vi "Multiple_DT98xx_Ain_Async_PN.vi"(7 "Master board name":string="DT9816(00)", 8 "Samples per channel":u32=2000, 9 "Sampling rate (Hz)":dbl=20000.0, 10 "Slave channels to acquire":string="0,1,2,3,4,5", 11 "Master channels to acquire":string="0,1,2,3,4,5") -> (0 "Overall error":errorcluster, 2 "Slaves data":dbl[][][](array[numeric]), 3 "Master data":dbl[][](graph))   [LabVIEW 2022 SP3]
uses:
  Low levels/DtAinContinuous Folder/PolySubVIs/DtCreateAinChan.vi
  Low levels/DtAinContinuous Folder/PolySubVIs/DtOLTimingSetInput.vi
  <userlib>/LV-Link3/PolySubVIs/DtOLStartNormal.vi
  Low levels/DtAinContinuous Folder/PolySubVIs/DtCreateCtrRateChan.vi
panel:
  out "Slaves data (concat.)":dbl[][](graph)
  out "Master board index":i32
  out "Board names":string[](array[string])=["DT9816(00)", "DT9816(01)"]
  out "Number of boards":i32=2
  # "DEVICES MUST BE INTERCONNECTED AS FOLLOWS:\nMaster \"Counter 0 Out\" to Master \"Ext Clock\" and Slaves \"Ext Clock\""
  # "PN 18/10/2012"
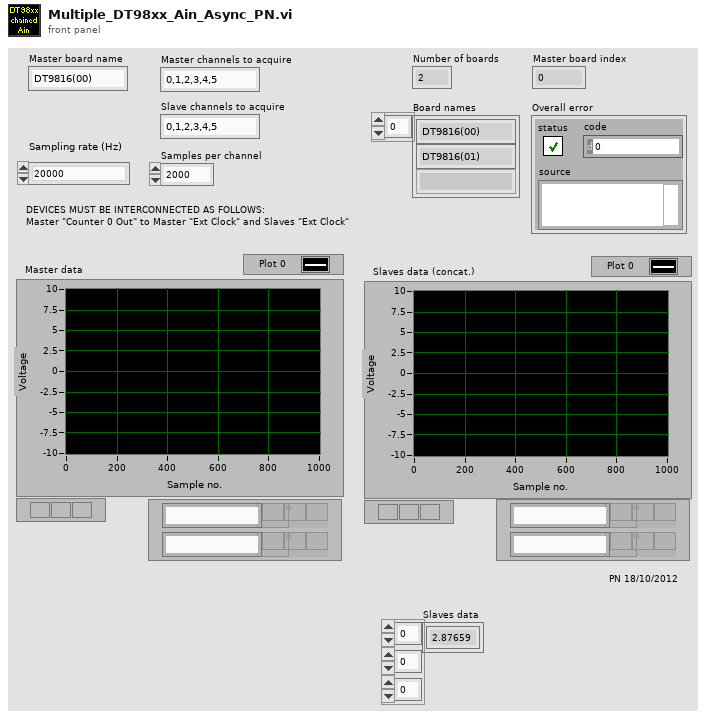
[diagram p1: front panel]
types:
  T1 = enum32{"Internal Clock", "External Clock", "No Timing"}
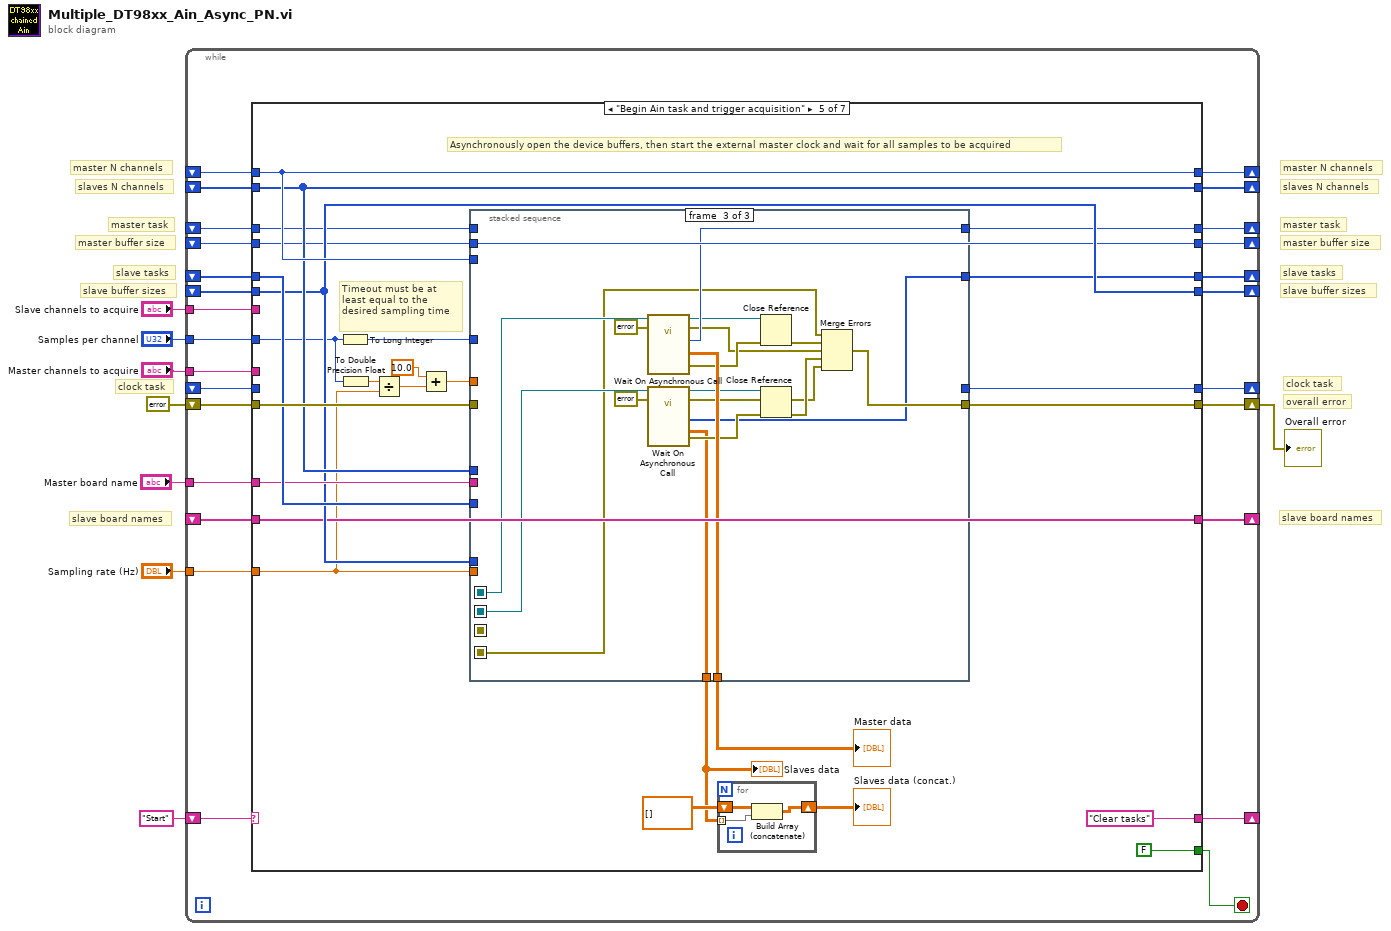
[diagram p0: block diagram]
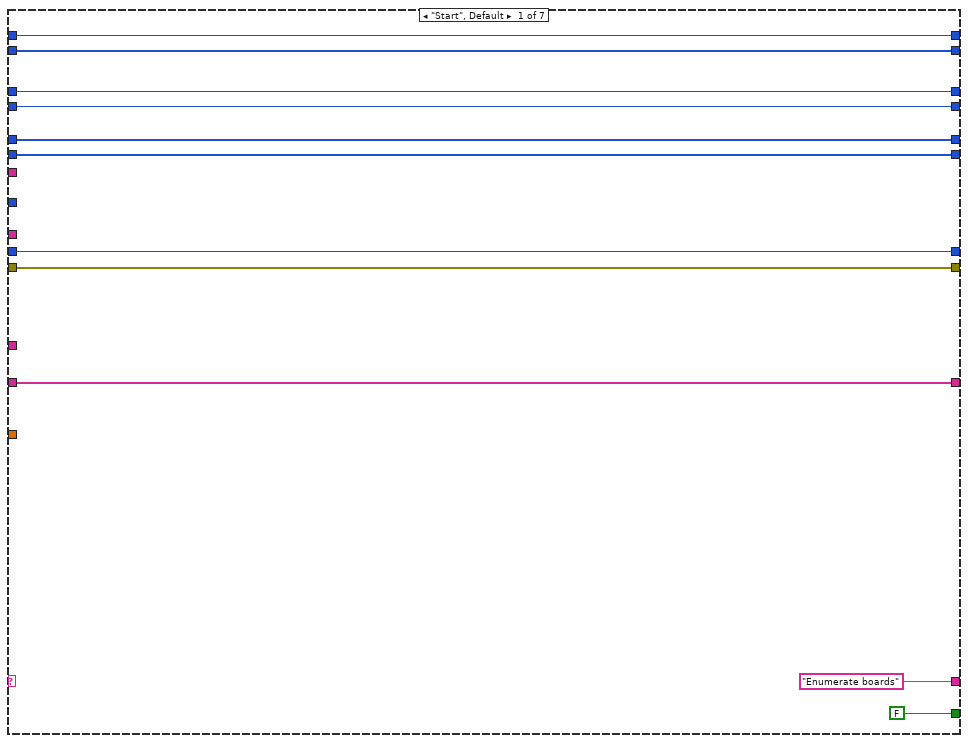
[diagram p2: hidden frame]
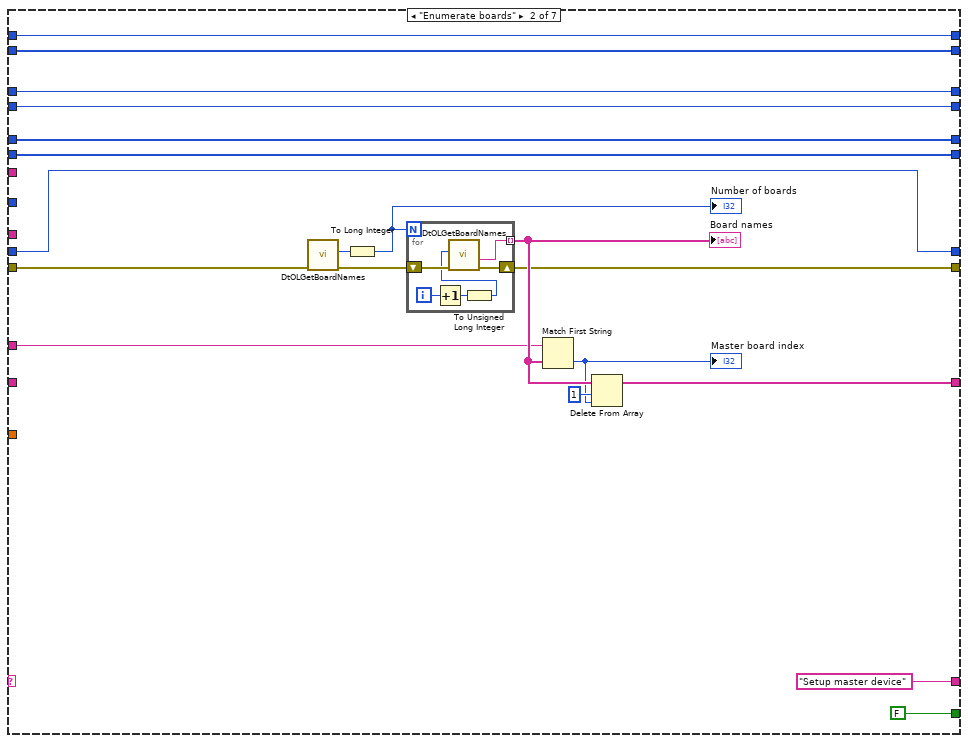
[diagram p3: hidden frame]
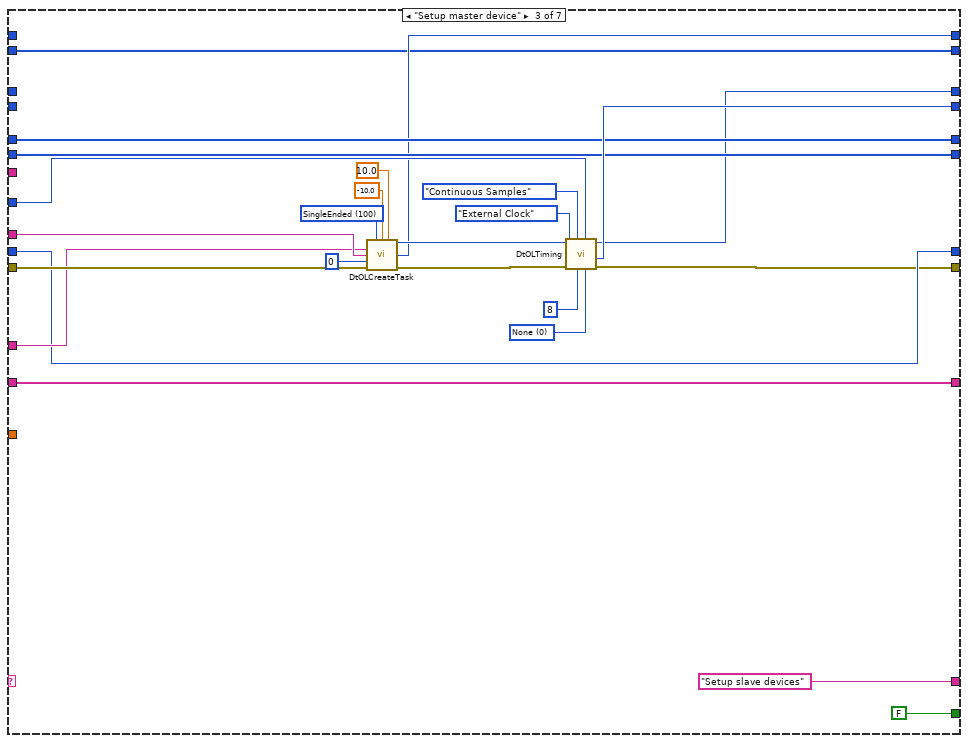
[diagram p4: hidden frame]
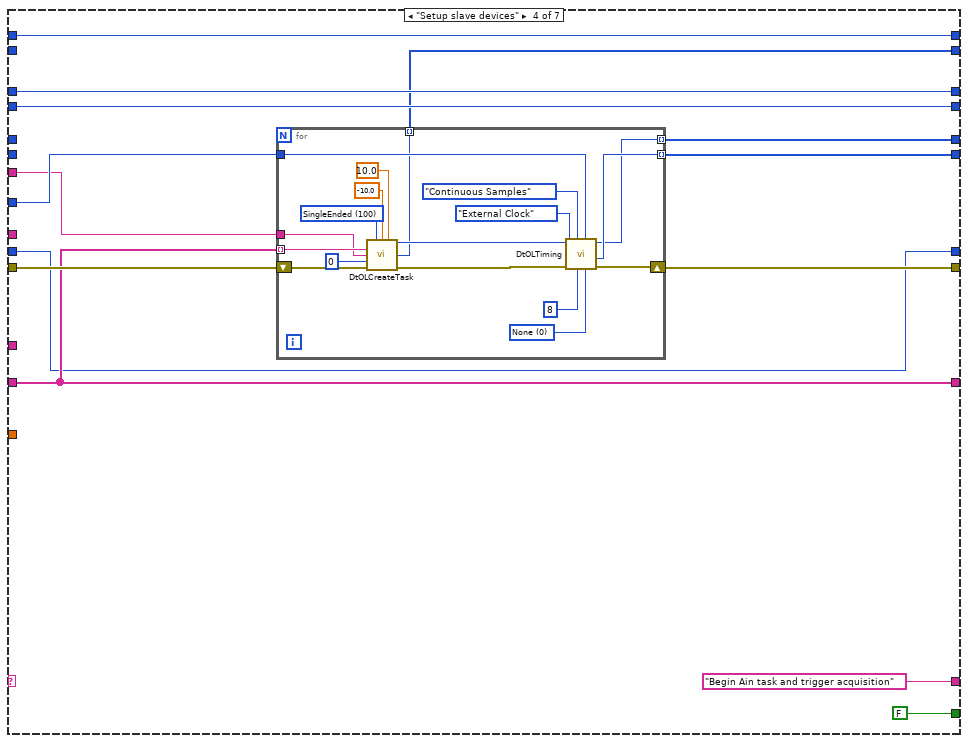
[diagram p5: hidden frame]
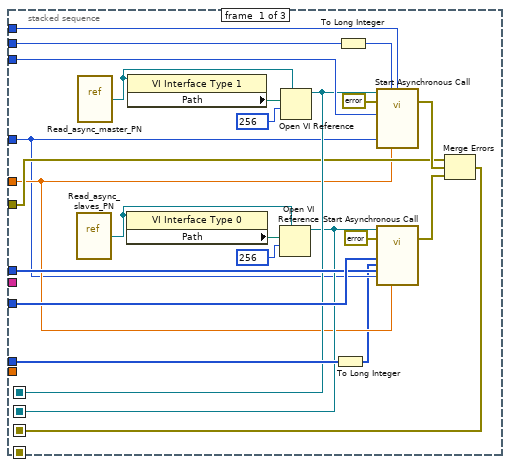
[diagram p6: hidden frame]
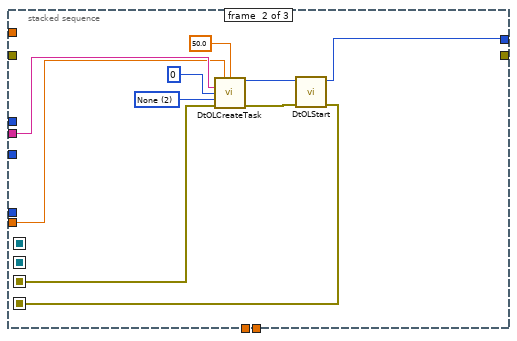
[diagram p7: hidden frame]
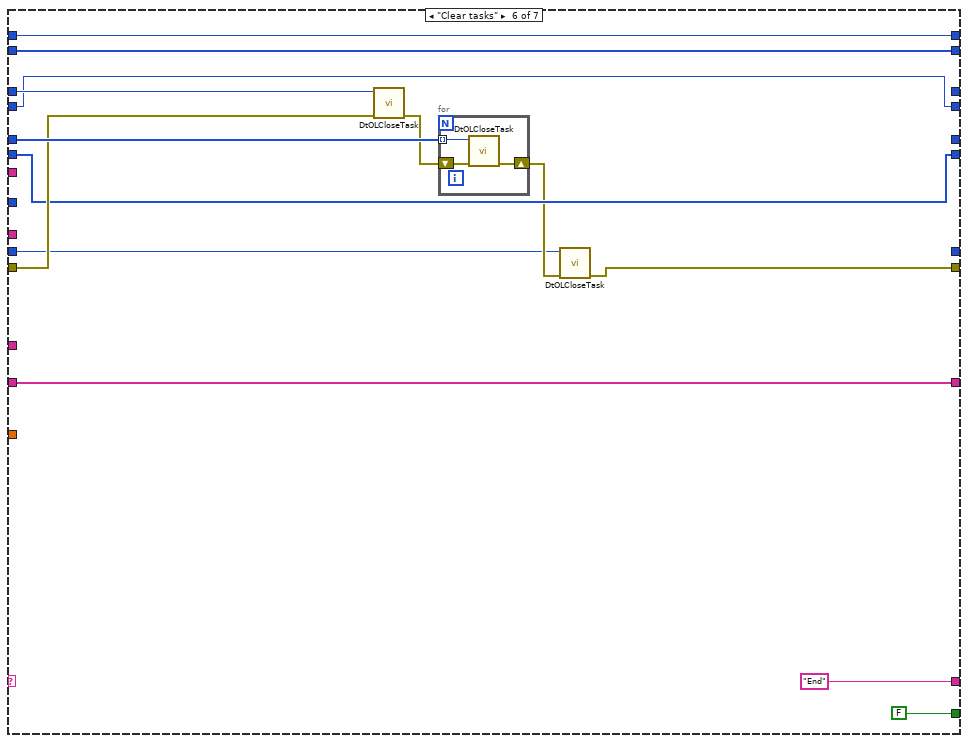
[diagram p8: hidden frame]
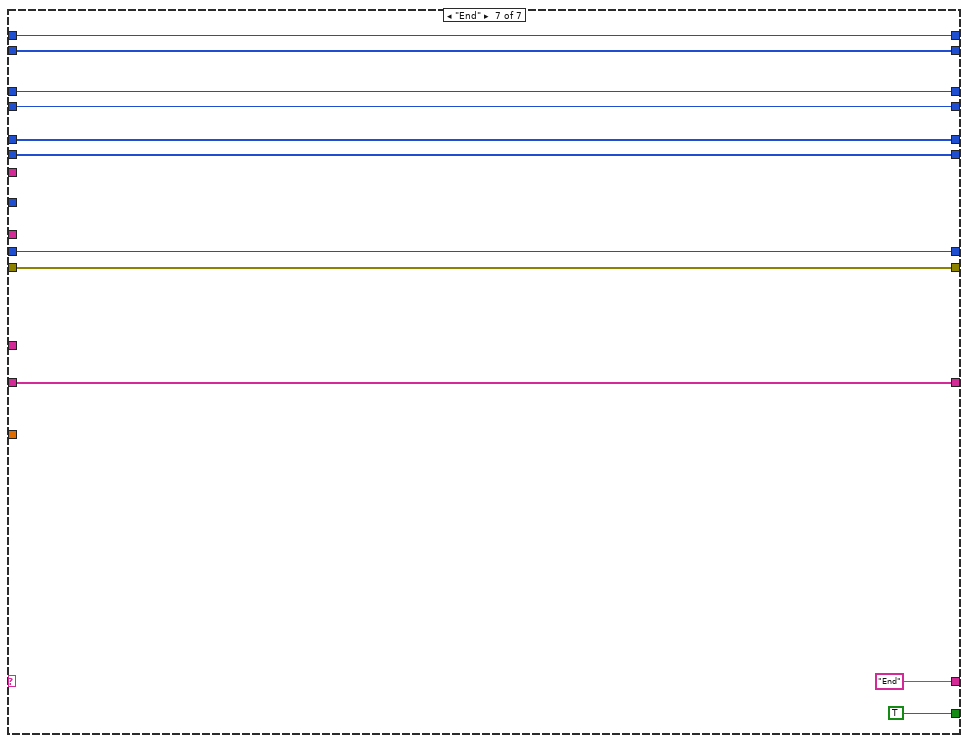
[diagram p9: hidden frame]
diagram:
  # "slave board names"
  # "clock task"
  # "slaves N channels"
  # "master N channels"
  # "master task"
  # "master buffer size"
  # "slave tasks"
  # "slave buffer sizes"
  # "overall error"
  # "clock task"
  # "slaves N channels"
  # "master N channels"
  # "master task"
  # "master buffer size"
  # "slave tasks"
  # "slave buffer sizes"
  # "slave board names"
  n1 = while {
    shift-right: [w32] -> _
    shift-left: "Start" -> [w33]
    shift-right: [w30] -> w1
    shift-left: errorcluster {"status"=FALSE, "code"=0, "source"=""} ("error in (no error)") -> [w31]
    shift-right: [w29] -> _
    shift-left: _ -> [w25]
    tunnel: "Master board name" -> [w28]
    tunnel: "Master channels to acquire" -> [w27]
    tunnel: "Samples per channel" -> [w26]
    shift-right: [w24] -> _
    shift-left: _ -> [w15]
    shift-right: [w23] -> _
    shift-left: _ -> [w14]
    shift-right: [w22] -> _
    shift-left: _ -> [w16]
    shift-right: [w21] -> _
    shift-left: _ -> [w17]
    shift-right: [w20] -> _
    shift-left: _ -> [w13]
    tunnel: "Sampling rate (Hz)" -> [w19]
    tunnel: "Slave channels to acquire" -> [w18]
    shift-right: [w12] -> _
    shift-left: _ -> [w9]
    shift-right: [w11] -> _
    shift-left: _ -> [w10]
    stop <- w34 stop-if-true
    n2 = case shown="\"Begin Ain task and trigger acquisition\"" w33 {
      tunnel: [FALSE FALSE FALSE FALSE FALSE FALSE TRUE] -> w34
      tunnel: ["Enumerate boards" "Setup master device" "Setup slave devices" "Begin Ain task and trigger acquisition" "Clear tasks" "End" "End"] -> w32
      tunnel: w31 -> [w38 w56 w81 w107 w151 w217 w227]
      tunnel: [w38 w55 w72 w106 w140 w210 w227] -> w30
      tunnel: [w37 w54 w78 w99 w143 w209 w226] -> w29
      tunnel: w28 -> [_ w53 w79 _ w149 _ _]
      tunnel: w27 -> [_ _ w80 _ _ _ _]
      tunnel: w26 -> [_ _ w83 w105 w134 _ _]
      tunnel: w25 -> [w37 _ w78 w99 w143 w209 w226]
      tunnel: [w41 w50 w76 w104 w136 _ w230] -> w24
      tunnel: [w40 w49 w75 w103 w146 w216 w229] -> w23
      tunnel: [w42 w51 w82 w100 w145 w215 w231] -> w22
      tunnel: [w43 w52 w71 w101 w137 _ w232] -> w21
      tunnel: [w39 w48 w77 w98 w135 _ w228] -> w20
      tunnel: w19 -> [_ _ _ _ w133 _ _]
      tunnel: w18 -> [_ _ _ w102 _ _ _]
      tunnel: w17 -> [w43 w52 _ w101 w144 w220 w232]
      tunnel: w16 -> [w42 w51 _ w100 w145 w215 w231]
      tunnel: w15 -> [w41 w50 w76 _ w150 w219 w230]
      tunnel: w14 -> [w40 w49 w75 _ w146 w216 w229]
      tunnel: w13 -> [w39 w48 w77 w98 _ w211 w228]
      tunnel: [w35 w46 w74 w96 w148 w214 w234] -> w12
      tunnel: [w36 w47 w73 w97 w147 w213 w233] -> w11
      tunnel: w10 -> [w36 w47 w73 _ w147 w213 w233]
      tunnel: w9 -> [w35 w46 _ w96 w148 w214 w234]
      frame "Start", Default {
      }
      frame "Enumerate boards" {
        n3 = call "DtOLGetBoardNames.vi"("error in (no error)"=w56) -> ("error out"=w60:errorcluster, "Number of boards"=w62:u32)  [unwired: 8 in, 1 out]
        n4 = To Long Integer(number=w62) -> (32bit integer=w61:i32)
        "Number of boards" <- w61
        n5 = for {
          N: w61 -> [_]
          shift-right: [w69] -> w55
          shift-left: w60 -> [w70]
          tunnel: [w68] -> w59 mode=indexing
          i -> [w67]
          n6 = Increment(x=w67) -> (x+1=w66:i32)
          n7 = To Unsigned Long Integer(number=w66) -> (unsigned 32bit integer=w65:u32)
          n8 = call "DtOLGetBoardNames.vi"("error in (no error)"=w70, "Select Board"=w65) -> ("error out"=w69:errorcluster, "Board Name"=w68:string)  [unwired: 7 in, 1 out]
        }
        "Board names" <- w59
        n9 = Match First String(2:w59, 3:w53) -> (0:w57:i32)  [unwired: 1 out]
        "Master board index" <- w57
        n10 = Delete From Array(array=w59, length=1, index=w57) -> (array with subset deleted=w54:string[])  [unwired: 1 out]
      }
      frame "Setup master device" {
        w84 = 0 items=["None", "Master", "Slave"] ("Sync Mode")
        w93 = 100 items=["SingleEnded"=100, "Differential"=101] ("Channel Type")
        n11 = call-poly "DtOLCreateTask.vi"("Channel Type"=w93, "Range Min"=-10.0, "Range Max"=10.0, "Board Name"=w79, "Channel"=w80, "Element"=u32 0, "error in (no error)"=w81) -> ("Task out"=w89:i32, "Actual Number of Channels"=w74:u32, "error out"=w88:errorcluster)  [unwired: 6 in]
        n12 = call-poly "DtOLTiming.vi"("Sync Mode"=w84, "Samples Per Channel"=w83, "Num Buffers"=u32 8, "Sample Mode"=enum16{"Finite Samples", "Continuous Samples"}."Continuous Samples", "error in (no error)"=w88, "Timing"=T1."External Clock", "Task in"=w89) -> ("error out"=w72:errorcluster, "Buffer Size"=w82:u32, "Task out"=w71:i32)  [unwired: 1 in, 1 out]
      }
      frame "Setup slave devices" {
        n13 = for {
          tunnel: w99 -> [w127] mode=indexing
          shift-right: [w110] -> w106
          shift-left: w107 -> [w125]
          tunnel: w102 -> [w123]
          tunnel: w105 -> [w116]
          tunnel: [w111] -> w104 mode=indexing
          tunnel: [w113] -> w103 mode=indexing
          tunnel: [w112] -> w97 mode=indexing
          w114 = 0 items=["None", "Master", "Slave"] ("Sync Mode")
          w126 = 100 items=["SingleEnded"=100, "Differential"=101] ("Channel Type")
          n14 = call-poly "DtOLCreateTask.vi"("Channel Type"=w126, "Range Min"=-10.0, "Range Max"=10.0, "Board Name"=w127, "Channel"=w123, "Element"=u32 0, "error in (no error)"=w125) -> ("Task out"=w120:i32, "Actual Number of Channels"=w112:u32, "error out"=w119:errorcluster)  [unwired: 6 in]
          n15 = call-poly "DtOLTiming.vi"("Sync Mode"=w114, "Samples Per Channel"=w116, "Num Buffers"=u32 8, "Sample Mode"=enum16{"Finite Samples", "Continuous Samples"}."Continuous Samples", "error in (no error)"=w119, "Timing"=T1."External Clock", "Task in"=w120) -> ("error out"=w110:errorcluster, "Buffer Size"=w113:u32, "Task out"=w111:i32)  [unwired: 1 in, 1 out]
        }
      }
      frame "Begin Ain task and trigger acquisition" {
        # "Timeout must be at least equal to the desired sampling time"
        # "Asynchronously open the device buffers, then start the external master clock and wait for all samples to be acquired"
        n16 = To Long Integer(number=w134) -> (32bit integer=w128:i32)
        n17 = To Double Precision Float(number=w134) -> (double precision float=w132:dbl)
        n18 = Divide(x=w132, y=w133) -> (x/y=w130:dbl)
        n19 = Add(x=10.0, y=w130) -> (x+y=w131:dbl)
        n20 = stacked-sequence {
          seq-local: [w167 _ _] -> [_ _ w192]
          seq-local: [w166 _ _] -> [_ _ w191]
          seq-local: [w161 _ _] -> [_ w180 _]
          seq-local: [_ w179 _] -> [_ _ w190]
          tunnel: w151 -> [w160 _ _]
          tunnel: w148 -> [w173 _ _]
          tunnel: w147 -> [w168 _ _]
          tunnel: w150 -> [w170 _ _]
          tunnel: w146 -> [w169 _ _]
          tunnel: w128 -> [w155 _ _]
          tunnel: w145 -> [w172 _ _]
          tunnel: w149 -> [_ w182 _]
          tunnel: w144 -> [w171 _ _]
          tunnel: [_ _ w205] -> w140
          tunnel: [_ _ w194] -> w139
          tunnel: [_ _ w204] -> w138
          tunnel: [_ _ w193] -> w136
          tunnel: [_ _ w203] -> w137
          tunnel: w133 -> [_ w181 _]
          tunnel: [_ w178 _] -> w135
          tunnel: w131 -> [w156 _ _]
          frame #0 {
            n21 = vi-ref "Read_async_slaves_PN.vi"() -> (w158:refnum<vi>)
            n22 = vi-ref "Read_async_master_PN.vi"() -> (w159:refnum<vi>)
            n23 = property class="VI Interface Type 0"(reference=w158) -> ("Path"=w175:path)  [unwired: 1 in, 2 out]
            n24 = property class="VI Interface Type 1"(reference=w159) -> ("Path"=w176:path)  [unwired: 1 in, 2 out]
            n25 = Open VI Reference(type specifier VI Refnum (for type only)=w158, vi path=w175, options=256) -> (vi reference=w166:refnum<vi>)  [unwired: 3 in, 1 out]
            n26 = Open VI Reference(type specifier VI Refnum (for type only)=w159, vi path=w176, options=256) -> (vi reference=w167:refnum<vi>)  [unwired: 3 in, 1 out]
            n27 = To Long Integer(number=w169) -> (32bit integer=w154:i32[])
            n28 = To Long Integer(number=w172) -> (32bit integer=w157:i32)
            n29 = call-by-ref "Start Asynchronous Call"(reference=w167, error in=errorcluster {"status"=FALSE, "code"=0, "source"=""} ("error in (no error)"), "master N channels"=w173, "master buffer size"=w157, "master task in"=w171, "Samples Per Channel"=w155, "Timeout"=w156) -> (error out=w165:errorcluster)  [unwired: 8 in, 4 out]
            n30 = call-by-ref "Start Asynchronous Call"(reference=w166, error in=errorcluster {"status"=FALSE, "code"=0, "source"=""} ("error in (no error)"), "slaves tasks"=w170, "slaves buffer sizes"=w154, "slave N channels"=w168, "Samples Per Channel"=w155, "Timeout"=w156) -> (error out=w164:errorcluster)  [unwired: 8 in, 4 out]
            n31 = Merge Errors(w160, w165, w164) -> (w161:errorcluster)
          }
          frame #1 {
            w186 = 2 items=["LowLevel", "HighLevel", "None"] ("Gate Type")
            n32 = call-poly "DtOLCreateTask.vi"("Requested\nFrequency (Hz)"=w181, "Duty Cycle"=50.0, "Board Name"=w182, "Counter Num"=u32 0, "Gate Type"=w186, "error in (no error)"=w180) -> ("Task out"=w184:i32, "error out"=w183:errorcluster)  [unwired: 7 in, 1 out]
            n33 = call-poly <userlib>:"DtOLStart.vi"("error in (no error)"=w183, "Task in"=w184) -> ("error out"=w179:errorcluster, "Task out"=w178:i32)  [unwired: 8 in]
          }
          frame #2 {
            n34 = call-by-ref "Wait On Asynchronous Call"(reference=w192, error in=errorcluster {"status"=FALSE, "code"=0, "source"=""} ("error in (no error)")) -> (reference out=w200:refnum<vi>, error out=w199:errorcluster, "master task out"=w203:i32, "master data"=w204:dbl[][], 15:"error out"=w202:errorcluster)  [unwired: 13 in]
            n35 = call-by-ref "Wait On Asynchronous Call"(reference=w191, error in=errorcluster {"status"=FALSE, "code"=0, "source"=""} ("error in (no error)")) -> (reference out=w198:refnum<vi>, error out=w195:errorcluster, "slaves tasks out"=w193:i32[], "slaves data"=w194:dbl[][][], 15:"error out"=w197:errorcluster)  [unwired: 13 in]
            n36 = Close Reference(reference=w200, error in (no error)=w202) -> (error out=w201:errorcluster)
            n37 = Close Reference(reference=w198, error in (no error)=w197) -> (error out=w196:errorcluster)
            n38 = Merge Errors(w190, w201, w199, w196, w195) -> (w205:errorcluster)
          }
        }
        "Master data" <- w138
        "Slaves data" <- w139
        n39 = for {
          shift-right: [w208] -> w142
          shift-left: dbl[][] [] -> [w207]
          tunnel: w139 -> [w206] mode=indexing
          n40 = Build Array (concatenate)(w207, w206) -> (w208:dbl[][])
        }
        "Slaves data (concat.)" <- w142
      }
      frame "Clear tasks" {
        n41 = call "DtOLCloseTask.vi"("Error in"=w217, "Task in"=w220) -> ("Error Out"=w218:errorcluster)  [unwired: 9 in]
        n42 = for {
          tunnel: w219 -> [w225] mode=indexing
          shift-right: [w223] -> w212
          shift-left: w218 -> [w224]
          n43 = call "DtOLCloseTask.vi"("Error in"=w224, "Task in"=w225) -> ("Error Out"=w223:errorcluster)  [unwired: 9 in]
        }
        n44 = call "DtOLCloseTask.vi"("Error in"=w212, "Task in"=w211) -> ("Error Out"=w210:errorcluster)  [unwired: 9 in]
      }
      frame "End" {
      }
    }
  }
  "Overall error" <- w1
